vi "2-15.vi"() -> ()   [LabVIEW 2022 SP3]
panel:
  in  "停止":bool
  out "颜色数值":i32 format="%x"
  in  "旋钮":i32(knob) scale=0.0..4.0 scale format="%x"
  out "波形图表":dbl(graph)
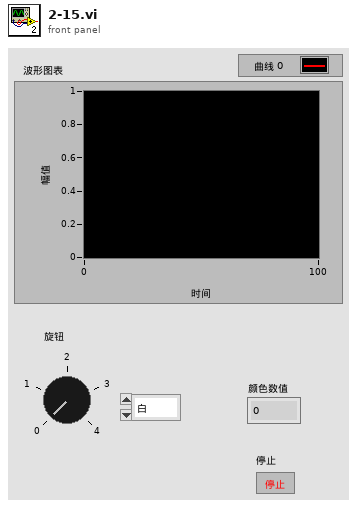
[diagram p1: front panel]
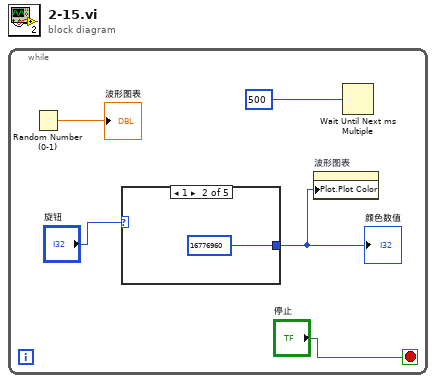
[diagram p0: block diagram]
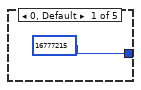
[diagram p2: hidden frame]
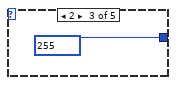
[diagram p3: hidden frame]
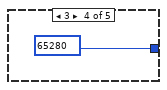
[diagram p4: hidden frame]
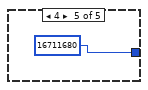
[diagram p5: hidden frame]
diagram:
  n1 = while {
    stop <- "停止" stop-if-true
    n2 = Random Number (0-1)() -> (number: 0 to 1=→"波形图表":dbl)
    n3 = case shown="1" "旋钮" {
      tunnel: [16777215 16776960 255 65280 16711680] -> w1
      frame 0, Default {
      }
      frame 1 {
      }
      frame 2 {
      }
      frame 3 {
      }
      frame 4 {
      }
    }
    "颜色数值" <- w1
    n4 = property on="波形图表" class="WFChart (严格)"("Plot.Plot Color"=w1) -> ()  [unwired: 2 in, 2 out]
    n5 = Wait Until Next ms Multiple(millisecond multiple=500) -> ()  [unwired: 1 out]
  }
